vi "SetAttribute.vi"(8 "error in (no error)":errorcluster, 10 "Set Attribute":T1, 11 "Data_Gaze in":refnum<class "Data_Gaze.lvclass">) -> (0 "error out":errorcluster, 3 "Data_Gaze out":refnum<class "Data_Gaze.lvclass">)   [LabVIEW 2020, in "Data_Gaze.lvclass"]
uses:
  Data_Gaze.lvclass
  Attribute.vi
  Data_Gaze.lvclass/Data_Gaze.ctl
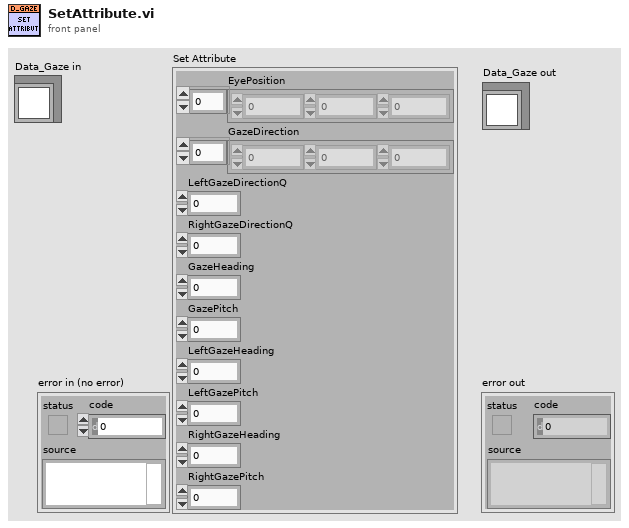
[diagram p1: front panel]
types:
  T1 = typedef "Data_Gaze.lvclass/Attribute.vi" = cluster{"EyePosition":dbl[], "GazeDirection":dbl[], "LeftGazeDirectionQ":dbl, "RightGazeDirectionQ":dbl, "GazeHeading":dbl, "GazePitch":dbl, "LeftGazeHeading":dbl, "LeftGazePitch":dbl, "RightGazeHeading":dbl, "RightGazePitch":dbl}
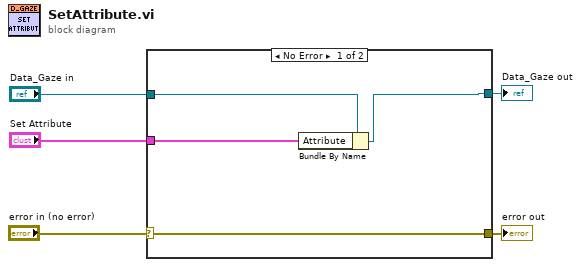
[diagram p0: block diagram]
diagram:
  n1 = case shown="No Error" "error in (no error)" {
    selector: "error in (no error)" -> [w9 w11]
    tunnel: [w9 w11] -> w4
    tunnel: [w7 w10] -> w3
    tunnel: "Data_Gaze in" -> [w8 w10]
    tunnel: "Set Attribute" -> [w6 _]
    frame No Error {
      n2 = Bundle By Name(cluster=w8, "Attribute"=w6) -> (w7:refnum<class "Data_Gaze.lvclass">)
    }
    frame Error {
    }
  }
  "error out" <- w4
  "Data_Gaze out" <- w3
